vi "动态数据.vi"() -> ()   [LabVIEW 2010]
uses:
  Instance           1 16Saved   动态数据 .vi
  Instance           2 16Saved   动态数据 .vi
  Instance           4 16Saved   动态数据 .vi
  <vilib>/Analysis/2dsp.llb/Power Spectrum (DBL).vi
  <vilib>/Analysis/NI_AALPro.lvlib
panel:
  out "Waveform Graph":dbl[](graph)
  out "Numeric":dbl
  out "Waveform Graph":dynamicdata(graph)
  out "Boolean":bool
  # "动 态 数 据 类 型"
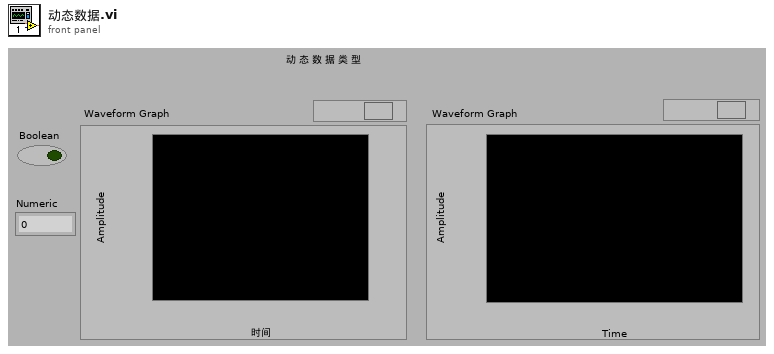
[diagram p1: front panel]
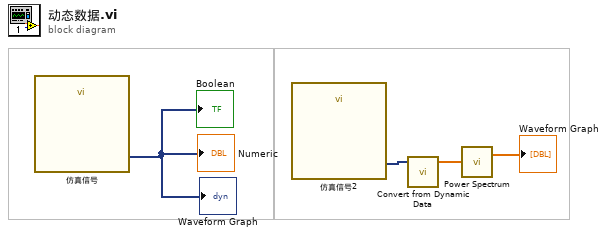
[diagram p0: block diagram]
diagram:
  n1 = call "仿真信号"() -> ("正弦"=→"Boolean" →"Waveform Graph" →"Numeric":dynamicdata)  [unwired: 14 in, 1 out]
  n2 = call "仿真信号2"() -> ("正弦"=w2:dynamicdata)  [unwired: 14 in, 1 out]
  n3 = call "Convert from Dynamic Data"("Dynamic Data Type"=w2) -> ("Array"=w3:dbl[])  [unwired: 3 in]
  n4 = call-poly <vilib>:"Power Spectrum.vi"("X"=w3) -> ("Power Spectrum"=→"Waveform Graph":dbl[])  [unwired: 1 out]
